vi "Mating.vi"() -> ()   [LabVIEW 2023]
uses:
  <vilib>/addons/database/Connection.llb/DB Tools Open Connec (String).vi
  <vilib>/regexp/Match Regular Expression.xnode
  <vilib>/addons/database/NI_Database_API.lvlib
panel:
  in  "Work Order":string
  in  "Exit":bool
  out "Sticker":bool
  out "Oscillator":bool
  out "Crystal":bool
  in  "Mating Type":string(combo)
  in  "Final DC_SN":string
  in  "Enter":bool
  in  "Crystal DC_SN":string
  in  "Base DC_SN":string
  # "DC_SN Mating Program"
  # "Please select mating type and\nenter needed information"
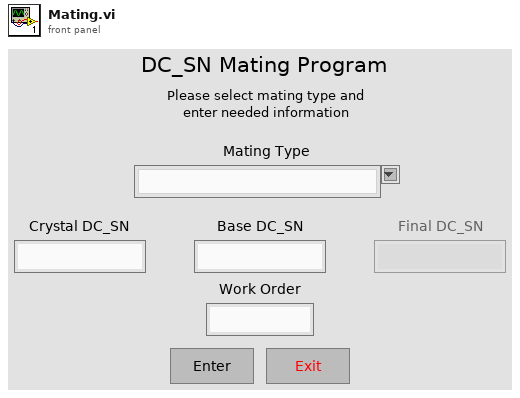
[diagram p1: front panel]
types:
  T1 = enum8{"Enabled", "Disabled", "Disabled and Grayed Out"}
  T2 = typedef "NI_Database_API.lvlib/Conn ObjectReference.ctl" = refnum<k1>
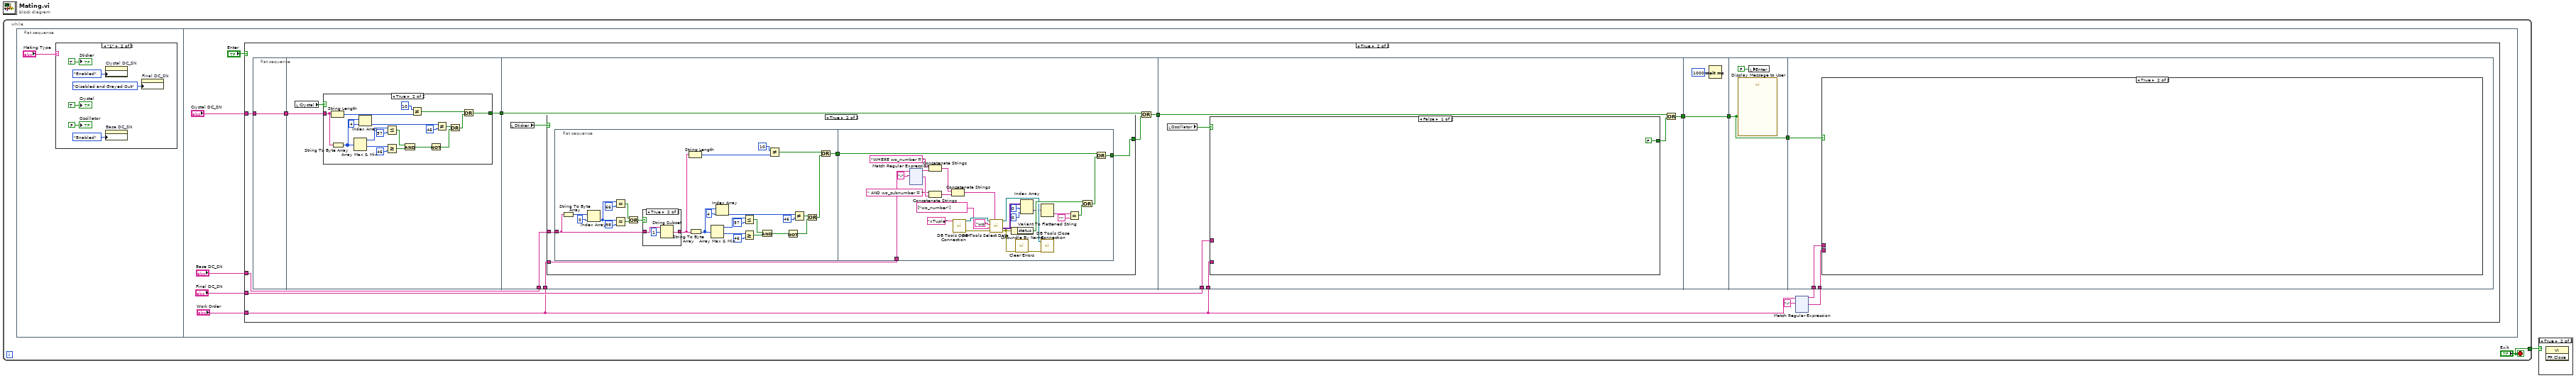
[diagram p0: block diagram]
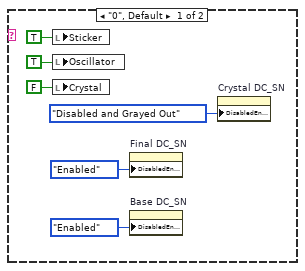
[diagram p3: hidden frame]
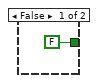
[diagram p5: hidden frame]
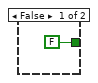
[diagram p6: hidden frame]
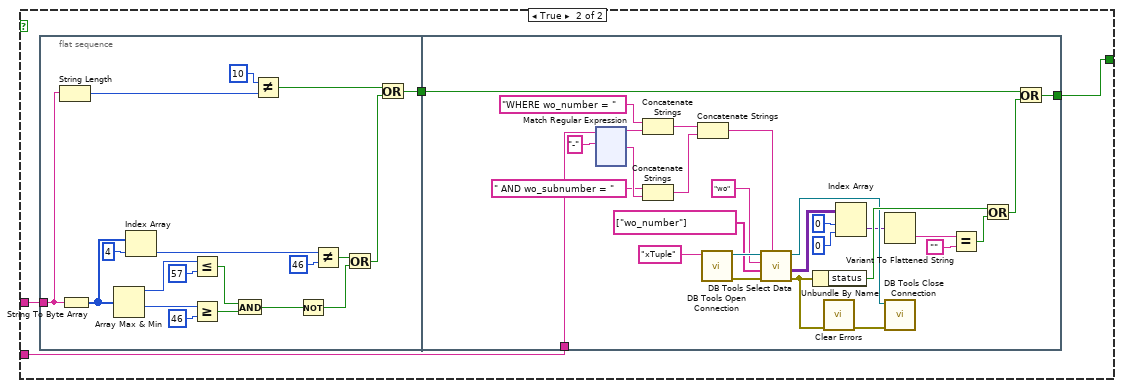
[diagram p8: hidden frame]
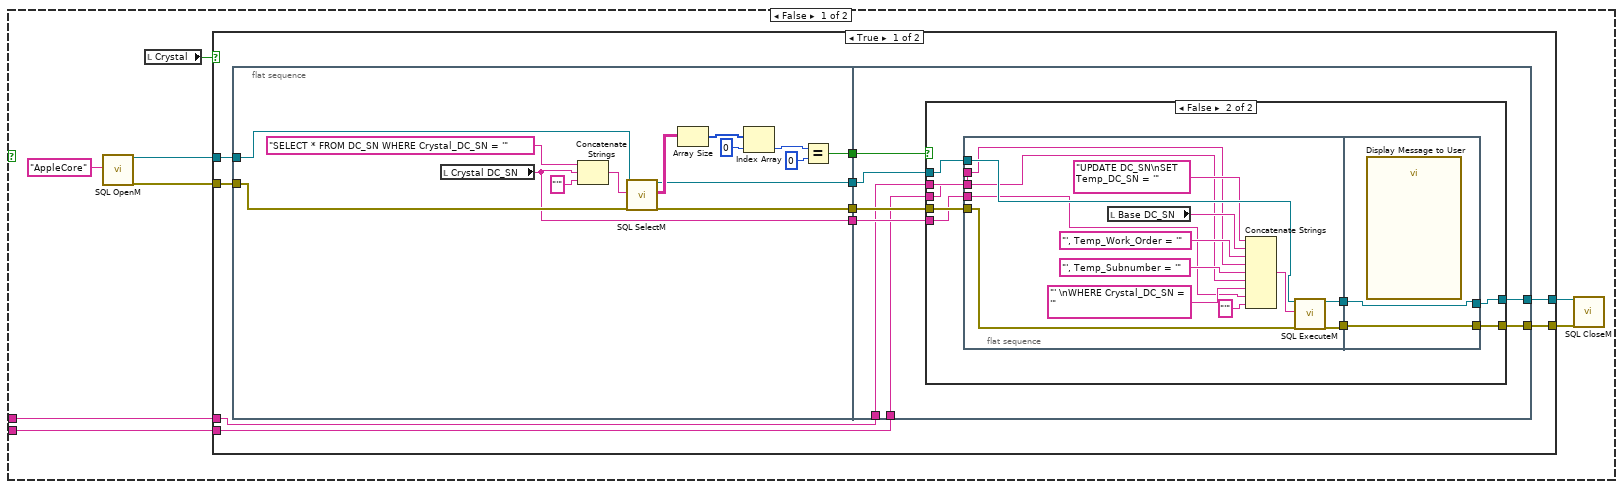
[diagram p9: hidden frame]
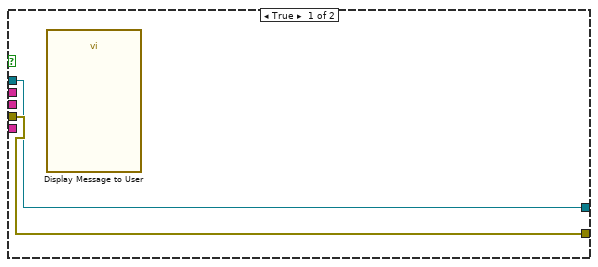
[diagram p10: hidden frame]
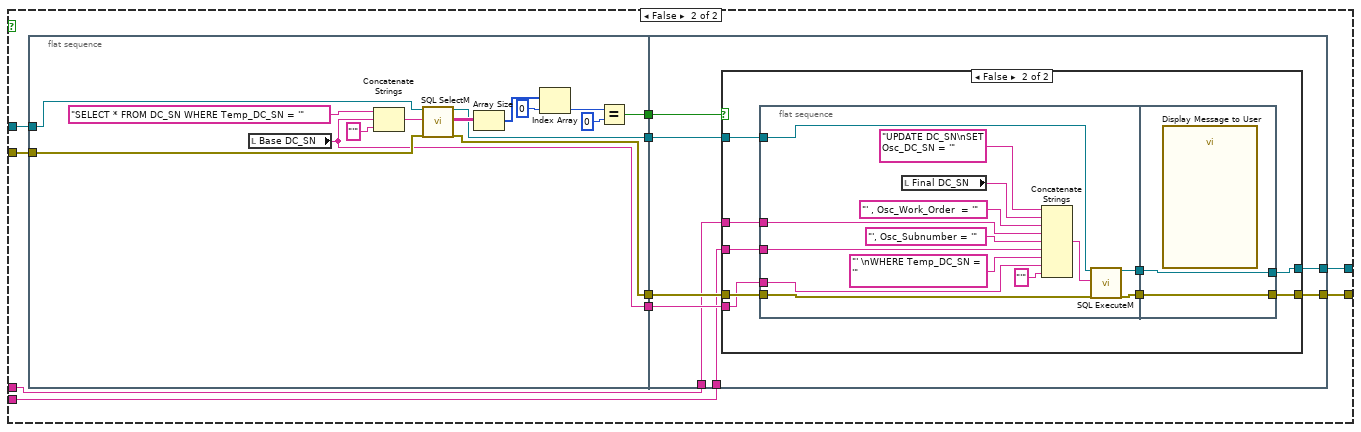
[diagram p11: hidden frame]
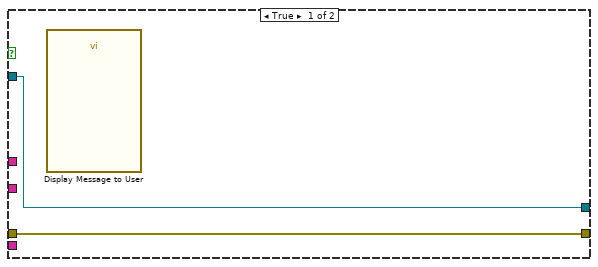
[diagram p12: hidden frame]
diagram:
  n1 = while {
    tunnel: ["Exit"] -> w1
    stop <- "Exit" stop-if-true
    n2 = flat-sequence {
      frame #0 {
        n3 = case shown="\"1\"" "Mating Type" {
          frame "0", Default {
            n4 = local write "Sticker"(TRUE ("Sticker")) -> ()
            n5 = local write "Oscillator"(TRUE ("Oscillator")) -> ()
            n6 = local write "Crystal"(FALSE ("Crystal")) -> ()
            n7 = property on="Final DC_SN" class="Str"("DisabledEnum"=T1."Enabled" ("Disabled")) -> ()  [unwired: 2 in, 2 out]
            n8 = property on="Base DC_SN" class="Str"("DisabledEnum"=T1."Enabled" ("Disabled")) -> ()  [unwired: 2 in, 2 out]
            n9 = property on="Crystal DC_SN" class="Str"("DisabledEnum"=T1."Disabled and Grayed Out" ("Disabled")) -> ()  [unwired: 2 in, 2 out]
          }
          frame "1" {
            n10 = property on="Crystal DC_SN" class="Str"("DisabledEnum"=T1."Enabled" ("Disabled")) -> ()  [unwired: 2 in, 2 out]
            n11 = property on="Base DC_SN" class="Str"("DisabledEnum"=T1."Enabled" ("Disabled")) -> ()  [unwired: 2 in, 2 out]
            n12 = property on="Final DC_SN" class="Str"("DisabledEnum"=T1."Disabled and Grayed Out" ("Disabled")) -> ()  [unwired: 2 in, 2 out]
            "Crystal" <- TRUE ("Crystal")
            "Oscillator" <- FALSE ("Oscillator")
            "Sticker" <- TRUE ("Sticker")
          }
        }
      }
      frame #1 {
        n13 = case shown="True" "Enter" {
          tunnel: "Crystal DC_SN" -> [_ w33]
          tunnel: "Base DC_SN" -> [_ w32]
          tunnel: "Final DC_SN" -> [_ w30]
          tunnel: "Work Order" -> [_ w21]
          frame False {
          }
          frame True {
            n14 = flat-sequence {
              tunnel: w33 -> [w151]
              tunnel: [w151] -> w27
              tunnel: [w153] -> w31
              tunnel: w27 -> [w154]
              tunnel: w32 -> [w177]
              tunnel: w31 -> [w176]
              tunnel: [w179] -> w29
              tunnel: w21 -> [w175]
              tunnel: w30 -> [w368]
              tunnel: w29 -> [w366]
              tunnel: [w365] -> w26
              tunnel: w21 -> [w363]
              tunnel: w26 -> [w539]
              tunnel: [w539] -> w25
              tunnel: w25 -> [w541]
              tunnel: [w541] -> w28
              tunnel: w28 -> [w544]
              tunnel: w23 -> [w543]
              tunnel: w22 -> [w542]
              frame #0 {
              }
              frame #1 {
                n15 = local read "Crystal"() -> (w152:bool)
                n16 = case shown="True" w152 {
                  tunnel: w154 -> [_ w157]
                  tunnel: [FALSE w156] -> w153
                  frame False {
                  }
                  frame True {
                    n17 = String Length(string=w157) -> (length=w174:i32)
                    n18 = String To Byte Array(string=w157) -> (unsigned byte array=w169:u8[])
                    n19 = Array Max & Min(array=w169) -> (max value=w167:u8, min value=w168:u8)  [unwired: 2 out]
                    n20 = Index Array(array=w169, index=4) -> (element=w172:u8)
                    n21 = Less Or Equal?(x=w167, y=u8 57) -> (x <= y?=w166:bool)
                    n22 = Greater Or Equal?(x=w168, y=u8 46) -> (x >= y?=w165:bool)
                    n23 = And(x=w166, y=w165) -> (x .and. y?=w164:bool)
                    n24 = Not Equal?(x=10, y=w174) -> (x != y?=w173:bool)
                    n25 = Not(x=w164) -> (.not. x?=w163:bool)
                    n26 = Not Equal?(x=w172, y=u8 46) -> (x != y?=w170:bool)
                    n27 = Or(x=w170, y=w163) -> (x .or. y?=w171:bool)
                    n28 = Or(x=w173, y=w171) -> (x .or. y?=w156:bool)
                  }
                }
              }
              frame #2 {
                n29 = local read "Sticker"() -> (w178:bool)
                n30 = case shown="True" w178 {
                  tunnel: [FALSE w184] -> w180
                  tunnel: w177 -> [_ w185]
                  tunnel: w175 -> [_ w182]
                  frame False {
                  }
                  frame True {
                    n31 = flat-sequence {
                      tunnel: w185 -> [w188]
                      tunnel: [w187] -> w183
                      tunnel: [w218] -> w184
                      tunnel: w183 -> [w219]
                      tunnel: w182 -> [w230]
                      frame #0 {
                        n32 = String To Byte Array(string=w188) -> (unsigned byte array=w190:u8[])
                        n33 = Index Array(array=w190, index=0) -> (element=w195:u8)
                        n34 = Equal?(x=w195, y=u8 66) -> (x = y?=w193:bool)
                        n35 = Equal?(x=w195, y=u8 98) -> (x = y?=w192:bool)
                        n36 = Or(x=w193, y=w192) -> (x .or. y?=w191:bool)
                        n37 = case shown="True" w191 {
                          tunnel: w188 -> [w214 w217]
                          tunnel: [w214 w215] -> w186
                          frame False {
                          }
                          frame True {
                            n38 = String Subset(string=w217, offset (0)=1) -> (substring=w215:string)  [unwired: 1 in]
                          }
                        }
                        n39 = String Length(string=w186) -> (length=w203:i32)
                        n40 = String To Byte Array(string=w186) -> (unsigned byte array=w189:u8[])
                        n41 = Array Max & Min(array=w189) -> (max value=w209:u8, min value=w208:u8)  [unwired: 2 out]
                        n42 = Index Array(array=w189, index=4) -> (element=w205:u8)
                        n43 = Less Or Equal?(x=w209, y=u8 57) -> (x <= y?=w210:bool)
                        n44 = Greater Or Equal?(x=w208, y=u8 46) -> (x >= y?=w211:bool)
                        n45 = And(x=w210, y=w211) -> (x .and. y?=w212:bool)
                        n46 = Not Equal?(x=10, y=w203) -> (x != y?=w204:bool)
                        n47 = Not(x=w212) -> (.not. x?=w213:bool)
                        n48 = Not Equal?(x=w205, y=u8 46) -> (x != y?=w207:bool)
                        n49 = Or(x=w207, y=w213) -> (x .or. y?=w206:bool)
                        n50 = Or(x=w204, y=w206) -> (x .or. y?=w187:bool)
                      }
                      frame #1 {
                        n51 = xnode "Match Regular Expression"("input string"=w230, "regular expression"="-") -> ("before match"=w244:string, "after match"=w245:string)  [unwired: 4 in, 3 out]
                        n52 = Concatenate Strings("WHERE wo_number = " ("string"), w244) -> (w234:string)
                        n53 = Concatenate Strings(" AND wo_subnumber = " ("string"), w245) -> (w235:string)
                        n54 = Concatenate Strings(w234, w235) -> (w236:string)
                        n55 = call-poly <vilib>:"DB Tools Open Connection.vi"("connection information"="xTuple" ("Connection Strings")) -> ("error out"=w243:errorcluster, "connection reference"=w242:T2)  [unwired: 7 in]
                        n56 = call <vilib>:"DB Tools Select Data.vi"("condition"=w236, "error in (no error)"=w243, "columns"=string[] ["wo_number"], "table"="wo", "connection reference"=w242) -> ("error out"=w238:errorcluster, "data"=w231:variant[][], "connection reference out"=w237:T2)  [unwired: 1 in]
                        n57 = Unbundle By Name(w238) -> ("status"=w241:bool)
                        n58 = call <vilib>:"Clear Errors.vi"("error in (no error)"=w238) -> ("error out"=w239:errorcluster)  [unwired: 5 in, 1 out]
                        n59 = Index Array(array=w231, index (row)=0, index (col)=0 ("disabled index (col)")) -> (element=w232:variant)
                        n60 = Variant To Flattened String(Variant=w232) -> (data string=w233:string)  [unwired: 1 out]
                        n61 = call <vilib>:"DB Tools Close Connection.vi"("error in (no error)"=w239, "connection reference"=w237) -> ()  [unwired: 5 in, 1 out]
                        n62 = Equal?(x=w233, y="") -> (x = y?=w240:bool)
                        n63 = Or(x=w241, y=w240) -> (x .or. y?=w220:bool)
                        n64 = Or(x=w219, y=w220) -> (x .or. y?=w218:bool)
                      }
                    }
                  }
                }
                n65 = Or(x=w176, y=w180) -> (x .or. y?=w179:bool)
              }
              frame #3 {
                n66 = local read "Oscillator"() -> (w364:bool)
                n67 = case shown="False" w364 {
                  tunnel: w368 -> [_ w373]
                  tunnel: [FALSE w372] -> w367
                  tunnel: w363 -> [_ w370]
                  frame False {
                  }
                  frame True {
                    n68 = flat-sequence {
                      tunnel: w373 -> [w375]
                      tunnel: [w374] -> w371
                      tunnel: [w393] -> w372
                      tunnel: w371 -> [w394]
                      tunnel: w370 -> [w395]
                      frame #0 {
                        n69 = String Length(string=w375) -> (length=w381:i32)
                        n70 = String To Byte Array(string=w375) -> (unsigned byte array=w386:u8[])
                        n71 = Array Max & Min(array=w386) -> (max value=w388:u8, min value=w387:u8)  [unwired: 2 out]
                        n72 = Index Array(array=w386, index=4) -> (element=w383:u8)
                        n73 = Less Or Equal?(x=w388, y=u8 57) -> (x <= y?=w389:bool)
                        n74 = Greater Or Equal?(x=w387, y=u8 46) -> (x >= y?=w390:bool)
                        n75 = And(x=w389, y=w390) -> (x .and. y?=w391:bool)
                        n76 = Not Equal?(x=10, y=w381) -> (x != y?=w382:bool)
                        n77 = Not(x=w391) -> (.not. x?=w392:bool)
                        n78 = Not Equal?(x=w383, y=u8 46) -> (x != y?=w385:bool)
                        n79 = Or(x=w385, y=w392) -> (x .or. y?=w384:bool)
                        n80 = Or(x=w382, y=w384) -> (x .or. y?=w374:bool)
                      }
                      frame #1 {
                        n81 = xnode "Match Regular Expression"("input string"=w395, "regular expression"="-") -> ("before match"=w419:string, "after match"=w420:string)  [unwired: 4 in, 3 out]
                        n82 = Concatenate Strings("WHERE wo_number = " ("string"), w419) -> (w409:string)
                        n83 = Concatenate Strings(" AND wo_subnumber = " ("string"), w420) -> (w410:string)
                        n84 = Concatenate Strings(w409, w410) -> (w411:string)
                        n85 = call-poly <vilib>:"DB Tools Open Connection.vi"("connection information"="xTuple" ("Connection Strings")) -> ("error out"=w418:errorcluster, "connection reference"=w417:T2)  [unwired: 7 in]
                        n86 = call <vilib>:"DB Tools Select Data.vi"("condition"=w411, "error in (no error)"=w418, "columns"=string[] ["wo_number"], "table"="wo", "connection reference"=w417) -> ("error out"=w413:errorcluster, "data"=w406:variant[][], "connection reference out"=w412:T2)  [unwired: 1 in]
                        n87 = Unbundle By Name(w413) -> ("status"=w416:bool)
                        n88 = call <vilib>:"Clear Errors.vi"("error in (no error)"=w413) -> ("error out"=w414:errorcluster)  [unwired: 5 in, 1 out]
                        n89 = Index Array(array=w406, index (row)=0, index (col)=0 ("disabled index (col)")) -> (element=w407:variant)
                        n90 = Variant To Flattened String(Variant=w407) -> (data string=w408:string)  [unwired: 1 out]
                        n91 = call <vilib>:"DB Tools Close Connection.vi"("error in (no error)"=w414, "connection reference"=w412) -> ()  [unwired: 5 in, 1 out]
                        n92 = Equal?(x=w408, y="") -> (x = y?=w415:bool)
                        n93 = Or(x=w416, y=w415) -> (x .or. y?=w396:bool)
                        n94 = Or(x=w394, y=w396) -> (x .or. y?=w393:bool)
                      }
                    }
                  }
                }
                n95 = Or(x=w366, y=w367) -> (x .or. y?=w365:bool)
              }
              frame #4 {
                n96 = Wait (ms)(milliseconds to wait=u32 1000) -> ()  [unwired: 1 out]
              }
              frame #5 {
                n97 = call "Display Message to User"("Enable"=w541) -> ()  [unwired: 9 in, 2 out]
                n98 = local write "Enter"(FALSE ("Enter")) -> ()
              }
              frame #6 {
                n99 = case shown="True" w544 {
                  tunnel: w543 -> [w546 _]
                  tunnel: w542 -> [w545 _]
                  frame False {
                    n100 = call "SQL OpenM.vi"("ConnectionString In"="AppleCore") -> ("Connection Out"=w551:refnum<k7>, "Error out"=w550:errorcluster)  [unwired: 17 in]
                    n101 = local read "Crystal"() -> (w547:bool)
                    n102 = case shown="True" w547 {
                      tunnel: w551 -> [w562 w621]
                      tunnel: w550 -> [w561 w620]
                      tunnel: [w560 w616] -> w549
                      tunnel: [w559 w615] -> w548
                      tunnel: w546 -> [w554 w613]
                      tunnel: w545 -> [w553 w612]
                      frame True {
                        n103 = flat-sequence {
                          tunnel: w562 -> [w576]
                          tunnel: w561 -> [w575]
                          tunnel: [w566] -> w558
                          tunnel: [w565] -> w557
                          tunnel: [w564] -> w556
                          tunnel: [w563] -> w555
                          tunnel: w558 -> [w584]
                          tunnel: w557 -> [w583]
                          tunnel: w556 -> [w582]
                          tunnel: w555 -> [w581]
                          tunnel: [w580] -> w560
                          tunnel: [w579] -> w559
                          tunnel: w554 -> [w578]
                          tunnel: w553 -> [w577]
                          frame #0 {
                            n104 = local read "Crystal DC_SN"() -> (w563:string)
                            n105 = Concatenate Strings("SELECT * FROM DC_SN WHERE Crystal_DC_SN = '" ("SQL Query"), w563, "'" ("string")) -> (w573:string)
                            n106 = call "SQL SelectM.vi"("Connection In"=w576, "SQL Query"=w573, "Error in (no error)"=w575) -> ("Connection Out"=w565:refnum<k7>, "Data"=w571:string[][], "Error out"=w564:errorcluster)  [unwired: 14 in]
                            n107 = Array Size(array=w571) -> (size(s)=w570:i32[])
                            n108 = Index Array(array=w570, index=0) -> (element=w568:i32)
                            n109 = Equal?(x=w568, y=0) -> (x = y?=w566:bool)
                          }
                          frame #1 {
                            n110 = case shown="False" w584 {
                              tunnel: w583 -> [w585 w595]
                              tunnel: w582 -> [w586 w594]
                              tunnel: [w585 w593] -> w580
                              tunnel: [w586 w592] -> w579
                              tunnel: w581 -> [_ w591]
                              tunnel: w578 -> [_ w588]
                              tunnel: w577 -> [_ w587]
                              frame True {
                                n111 = call "Display Message to User"() -> ()  [unwired: 10 in, 2 out]
                              }
                              frame False {
                                n112 = flat-sequence {
                                tunnel: w595 -> [w609]
                                tunnel: w594 -> [w608]
                                tunnel: w591 -> [w597]
                                tunnel: [w607] -> w590
                                tunnel: [w606] -> w589
                                tunnel: w588 -> [w601]
                                tunnel: w587 -> [w599]
                                tunnel: [w610] -> w592
                                tunnel: [w611] -> w593
                                tunnel: w590 -> [w611]
                                tunnel: w589 -> [w610]
                                frame #0 {
                                n113 = local read "Base DC_SN"() -> (w603:string)
                                n114 = Concatenate Strings("UPDATE DC_SN\nSET Temp_DC_SN = '" ("SQL Query"), w603, "', Temp_Work_Order = '" ("string"), w601, "', Temp_Subnumber = '" ("string"), w599, "' \nWHERE Crystal_DC_SN = '" ("string"), w597, "'" ("string")) -> (w604:string)
                                n115 = call "SQL ExecuteM.vi"("Connection In"=w609, "SQL Query"=w604, "Error in (no error)"=w608) -> ("Connection Out"=w607:refnum<k7>, "Error out"=w606:errorcluster)  [unwired: 15 in]
                                }
                                frame #1 {
                                n116 = call "Display Message to User"() -> ()  [unwired: 10 in, 2 out]
                                }
                                }
                              }
                            }
                          }
                        }
                      }
                      frame False {
                        n117 = flat-sequence {
                          tunnel: w621 -> [w635]
                          tunnel: w620 -> [w634]
                          tunnel: [w625] -> w619
                          tunnel: [w624] -> w618
                          tunnel: [w623] -> w617
                          tunnel: [w622] -> w614
                          tunnel: w619 -> [w643]
                          tunnel: w618 -> [w642]
                          tunnel: w617 -> [w641]
                          tunnel: [w640] -> w616
                          tunnel: [w639] -> w615
                          tunnel: w614 -> [w638]
                          tunnel: w613 -> [w637]
                          tunnel: w612 -> [w636]
                          frame #0 {
                            n118 = local read "Base DC_SN"() -> (w622:string)
                            n119 = Concatenate Strings("SELECT * FROM DC_SN WHERE Temp_DC_SN = '" ("SQL Query"), w622, "'" ("string")) -> (w632:string)
                            n120 = call "SQL SelectM.vi"("Connection In"=w635, "SQL Query"=w632, "Error in (no error)"=w634) -> ("Connection Out"=w624:refnum<k7>, "Data"=w630:string[][], "Error out"=w623:errorcluster)  [unwired: 14 in]
                            n121 = Array Size(array=w630) -> (size(s)=w629:i32[])
                            n122 = Index Array(array=w629, index=0) -> (element=w627:i32)
                            n123 = Equal?(x=w627, y=0) -> (x = y?=w625:bool)
                          }
                          frame #1 {
                            n124 = case shown="False" w643 {
                              tunnel: w642 -> [w645 w654]
                              tunnel: w641 -> [w644 w653]
                              tunnel: [w645 w652] -> w640
                              tunnel: [w644 w651] -> w639
                              tunnel: w638 -> [_ w650]
                              tunnel: w637 -> [_ w647]
                              tunnel: w636 -> [_ w646]
                              frame True {
                                n125 = call "Display Message to User"() -> ()  [unwired: 10 in, 2 out]
                              }
                              frame False {
                                n126 = flat-sequence {
                                tunnel: w654 -> [w668]
                                tunnel: w653 -> [w667]
                                tunnel: w650 -> [w655]
                                tunnel: [w666] -> w649
                                tunnel: [w665] -> w648
                                tunnel: w647 -> [w661]
                                tunnel: w646 -> [w658]
                                tunnel: [w669] -> w651
                                tunnel: [w670] -> w652
                                tunnel: w649 -> [w670]
                                tunnel: w648 -> [w669]
                                frame #0 {
                                n127 = local read "Final DC_SN"() -> (w662:string)
                                n128 = Concatenate Strings("UPDATE DC_SN\nSET Osc_DC_SN = '" ("SQL Query"), w662, "' , Osc_Work_Order  = '" ("string"), w661, "', Osc_Subnumber = '" ("string"), w658, "' \nWHERE Temp_DC_SN = '" ("string"), w655, "'" ("string")) -> (w663:string)
                                n129 = call "SQL ExecuteM.vi"("Connection In"=w668, "SQL Query"=w663, "Error in (no error)"=w667) -> ("Connection Out"=w666:refnum<k7>, "Error out"=w665:errorcluster)  [unwired: 15 in]
                                }
                                frame #1 {
                                n130 = call "Display Message to User"() -> ()  [unwired: 10 in, 2 out]
                                }
                                }
                              }
                            }
                          }
                        }
                      }
                    }
                    n131 = call "SQL CloseM.vi"("Connection In"=w549, "Error in (no error)"=w548) -> ()  [unwired: 17 in, 1 out]
                  }
                  frame True {
                  }
                }
              }
            }
            n132 = xnode "Match Regular Expression"("input string"=w21, "regular expression"="-") -> ("before match"=w23:string, "after match"=w22:string)  [unwired: 4 in, 3 out]
          }
        }
      }
    }
  }
  n133 = case shown="True" w1 {
    frame False {
    }
    frame True {
      n134 = invoke class="VI" method="FP.Close"() -> ()  [unwired: 3 in, 3 out]
    }
  }
